vi "HandleInput.vi"(8 "error in (no error)":errorcluster, 10 "TeleopInstruction":T1) -> (0 "error out":errorcluster)   [LabVIEW 2013]
uses:
  KariQueue/TeleopInstruction.ctl
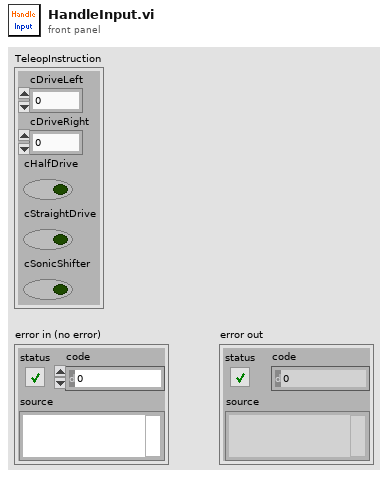
[diagram p1: front panel]
types:
  T1 = typedef "TeleopInstruction.ctl" = cluster{"cDriveLeft":dbl, "cDriveRight":dbl, "cHalfDrive":bool, "cStraightDrive":bool, "cSonicShifter":bool}
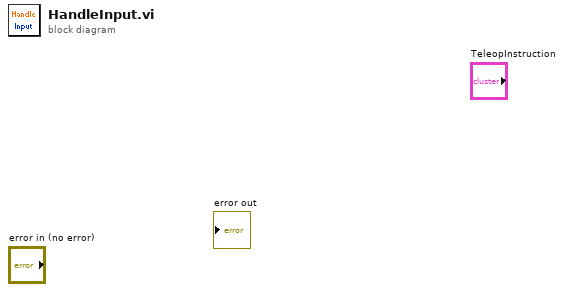
[diagram p0: block diagram]
diagram:
